vi "Pulse Debounce & Delay.vi"(1 "Delay (sec)":dbl, 2 "In":bool, 4 "Width (sec)":dbl=0.01) -> (5 "Out":bool)   [LabVIEW 2013]
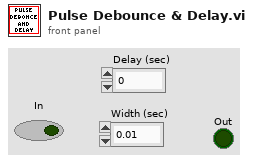
[diagram p1: front panel]
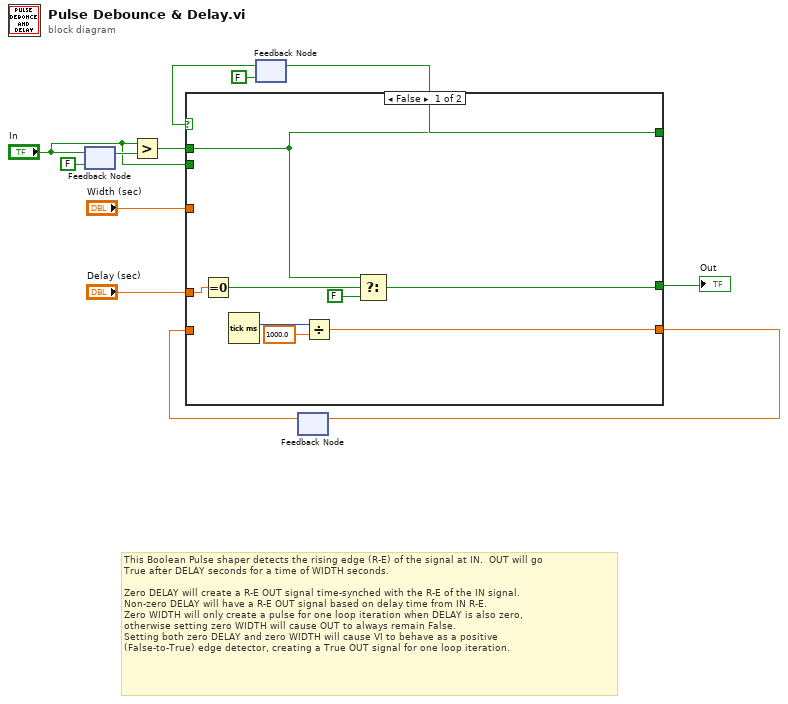
[diagram p0: block diagram]
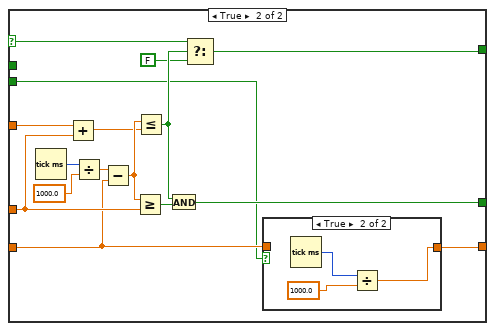
[diagram p2: hidden frame]
diagram:
  # "This Boolean Pulse shaper detects the rising edge (R-E) of the signal at IN.  OUT will go\nTrue after DELAY seconds for a time of WIDTH seconds. \n\nZero DELAY will create a R-E OUT signal time-synched with the R-E of the IN signal.\nNon-zero DELAY will have a R-E OUT signal based on delay time from IN R-E.\nZero WIDTH will only create a pulse for one loop iteration when DELAY is also zero,\notherwise setting zero WIDTH will cause OUT to always remain False.\nSetting both zero DELAY and zero WIDTH will cause VI to behave as a positive\n(False-to-True) edge detector, creating a True OUT signal for one loop iteration."
  n1 = feedback #1(FALSE ("input")) -> (w11:bool)
  n2 = feedback-in #1("In") -> ()
  n3 = Greater?(x="In", y=w11) -> (0:w3:bool)
  n4 = feedback #2(FALSE) -> (w7:bool)
  n5 = feedback #3() -> (w9:dbl)  [unwired: 1 in]
  n6 = case shown="False" w7 {
    selector: w7 -> [_ w30]
    tunnel: [w13 w22] -> w10
    tunnel: w9 -> [_ w23]
    tunnel: [w19 w36] -> w8
    tunnel: w3 -> [w19 _]
    tunnel: [w18 w34] -> w2
    tunnel: "Delay (sec)" -> [w20 w28]
    tunnel: "Width (sec)" -> [_ w27]
    tunnel: "In" -> [_ w21]
    frame False {
      n7 = Equal To 0?(x=w20) -> (x = 0?=w16:bool)
      n8 = Tick Count (ms)() -> (millisecond timer value=w15:u32)
      n9 = Divide(x=w15, y=1000.0) -> (x/y=w13:dbl)
      n10 = Select(t=w19, s=w16, f=FALSE) -> (s? t:f=w18:bool)
    }
    frame True {
      n11 = Tick Count (ms)() -> (millisecond timer value=w25:u32)
      n12 = Add(x=w27, y=w28) -> (x+y=w32:dbl)
      n13 = Divide(x=w25, y=1000.0) -> (x/y=w26:dbl)
      n14 = Subtract(x=w26, y=w23) -> (x-y=w33:dbl)
      n15 = Greater Or Equal?(x=w33, y=w28) -> (x >= y?=w35:bool)
      n16 = Less Or Equal?(x=w33, y=w32) -> (x <= y?=w31:bool)
      n17 = And(x=w31, y=w35) -> (x .and. y?=w34:bool)
      n18 = Select(t=w30, s=w31, f=FALSE) -> (s? t:f=w36:bool)
      n19 = case shown="True" w21 {
        tunnel: [w37 w38] -> w22
        tunnel: w23 -> [w37 _]
        frame False {
        }
        frame True {
          n20 = Tick Count (ms)() -> (millisecond timer value=w40:u32)
          n21 = Divide(x=w40, y=1000.0) -> (x/y=w38:dbl)
        }
      }
    }
  }
  "Out" <- w2
  n22 = feedback-in #2(w8) -> ()
  n23 = feedback-in #3(w10) -> ()
